vi "rotBendingMode.vi"(8 "error in (no error)":errorcluster, 9 "Tilt Angle (arcsec)":cluster{"Tile X":dbl, "Tilt Y":dbl}, 10 "Mirror DOF (um)":dbl[](array[numeric]), 11 "CamRot in":refnum<class "CamRot.lvclass">) -> (0 "error out":errorcluster, 2 "Rotated Mirror DOF (um)":dbl[](array[numeric]), 3 "CamRot out":refnum<class "CamRot.lvclass">)   [LabVIEW 2016, in "OfcFunc.lvlib" / "CamRot.lvclass"]
doc: "Rotate the bending mode (degree of freedom, DOF) based on the rotation angle and tilt angle compared with the camera."
uses:
  CamRot.lvclass
  CamRot.lvclass/CamRot.ctl
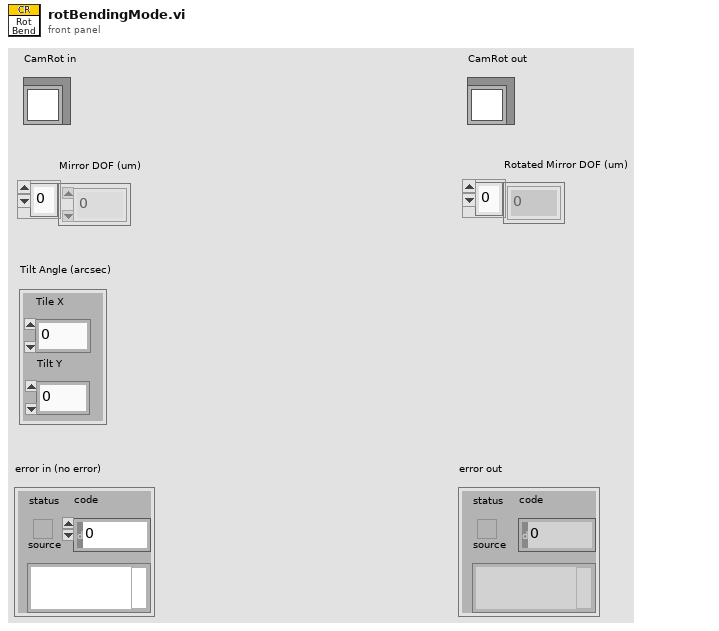
[diagram p1: front panel]
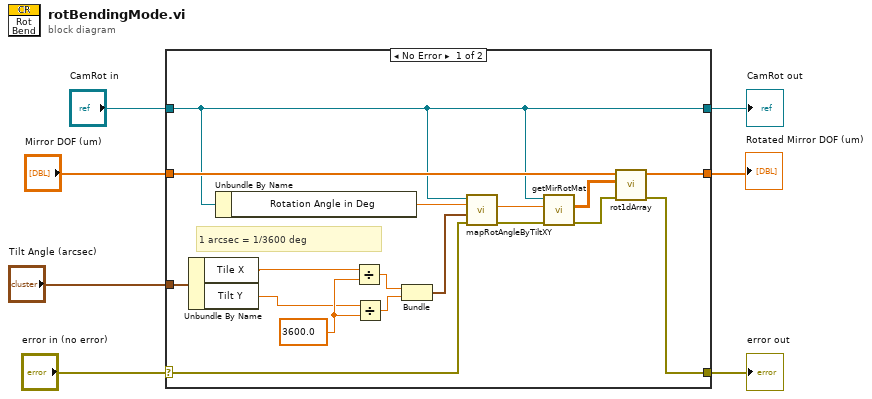
[diagram p0: block diagram]
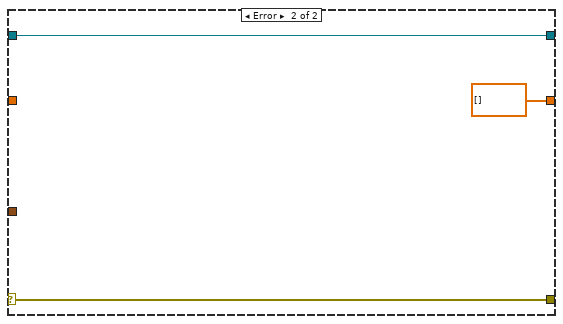
[diagram p2: hidden frame]
diagram:
  n1 = case shown="No Error" "error in (no error)" {
    selector: "error in (no error)" -> [w10 w27]
    tunnel: [w21 w27] -> w6
    tunnel: [w13 w26] -> w4
    tunnel: "CamRot in" -> [w13 w26]
    tunnel: "Mirror DOF (um)" -> [w24 _]
    tunnel: [w20 dbl[] [] ("Rotated 1D Array")] -> w2
    tunnel: "Tilt Angle (arcsec)" -> [w19 _]
    frame No Error {
      w18 = 3600.0
      # "1 arcsec = 1/3600 deg"
      n2 = Unbundle By Name(w19) -> ("Tile X"=w15:dbl, "Tilt Y"=w14:dbl)
      n3 = Unbundle By Name(w13) -> ("Rotation Angle in Deg"=w12:dbl)
      n4 = Divide(x=w15, y=w18) -> (x/y=w17:dbl)
      n5 = Divide(x=w14, y=w18) -> (x/y=w16:dbl)
      n6 = Bundle(w17, w16) -> (w11:cluster{dbl, dbl})  [unwired: 1 in]
      n7 = call "mapRotAngleByTiltXY.vi"("error in (no error)"=w10, "Tilt Angle (degree)"=w11, "Rotation Angle in Deg"=w12, "CamRot in"=w13) -> ("error out"=w9:errorcluster, "Mapped Rotation Angle in Deg"=w8:dbl)  [unwired: 5 in, 1 out]
      n8 = call "getMirRotMat.vi"("error in (no error)"=w9, "Rotation Angle in Deg"=w8, "CamRot in"=w13) -> ("error out"=w22:errorcluster, "Rotation Matrix"=w23:dbl[][])  [unwired: 6 in, 1 out]
      n9 = call "rot1dArray.vi"("error in (no error)"=w22, "Rot Mat"=w23, "1D Array"=w24) -> ("error out"=w21:errorcluster, "Rotated 1D Array"=w20:dbl[])  [unwired: 7 in]
    }
    frame Error {
    }
  }
  "error out" <- w6
  "CamRot out" <- w4
  "Rotated Mirror DOF (um)" <- w2
